vi "ep_Check Range of Rated Speed.vi"(8 "error in (no error)":errorcluster, 10 "speed [RPM]":dbl, 11 "nominal frequency":enum16{"50 Hz", "60 Hz"}(ring)) -> (0 "error out":errorcluster)   [LabVIEW 2014, in "NI_EP_Motor Monitoring.lvlib"]
uses:
  <vilib>/addons/Electrical Power/Motor Monitoring/NI_EP_Motor Monitoring.lvlib
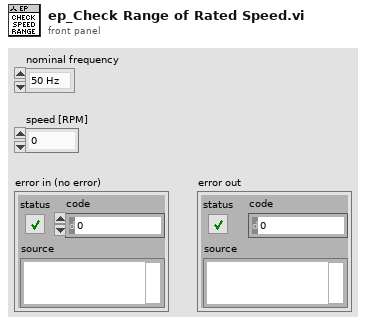
[diagram p1: front panel]
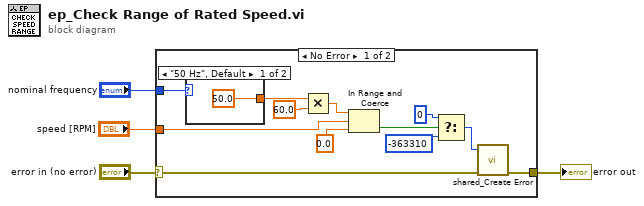
[diagram p0: block diagram]
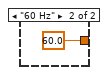
[diagram p2: hidden frame]
diagram:
  n1 = case shown="No Error" "error in (no error)" {
    selector: "error in (no error)" -> [w6 w19]
    tunnel: "nominal frequency" -> [w9 _]
    tunnel: "speed [RPM]" -> [w8 _]
    tunnel: [w5 w19] -> w1
    frame No Error {
      n2 = case shown="\"50 Hz\", Default" w9 {
        tunnel: [50.0 60.0] -> w11
        frame "50 Hz", Default {
        }
        frame "60 Hz" {
        }
      }
      n3 = Multiply(x=w11, y=60.0) -> (x*y=w10:dbl)
      n4 = In Range and Coerce(upper limit=w10, x=w8, lower limit=0.0 ("upper limit")) -> (In Range?=w7:bool)  [unwired: 1 out]
      n5 = Select(t=0 ("y"), s=w7, f=-363310 ("y")) -> (s? t:f=w14:i32)
      n6 = call <vilib>:"shared_Create Error.vi"("error in (no error)"=w6, "error code (0)"=w14) -> ("error out"=w5:errorcluster)  [unwired: 9 in]
    }
    frame Error {
    }
  }
  "error out" <- w1
